vi "AMZ_S3_APIHLP_Multipart Upload Data FG - Get.vi"(8 "error in (no error)":errorcluster, 11 "Multipart Upload RefNum in":T3) -> (0 "error out":errorcluster, 2 "Multipart Upload Data":T1 {"Parts"."PartNumber" min=1 max=10000}, 3 "Multipart Upload RefNum out":T3)   [LabVIEW 2015, in "LV Interface for Amazon S3.lvlib"]
uses:
  LV Interface for Amazon S3.lvlib
  Typedefs/AMZ_S3_Multipart Upload RefNum.ctl
  Typedefs/AMZ_S3_Multipart Upload RefNum Enum.ctl
  Typedefs/AMZ_S3_Multipart Upload Data.ctl
  Typedefs/AMZ_S3_Multipart Upload Part Data.ctl
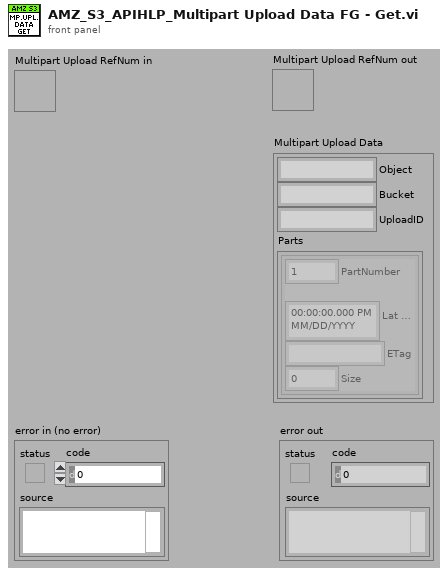
[diagram p1: front panel]
types:
  T1 = typedef "LV Interface for Amazon S3.lvlib/AMZ_S3_Multipart Upload Data.ctl" = cluster{"Object":string, "Bucket":string, "UploadID":string, "Parts":T2[]}
  T2 = typedef "LV Interface for Amazon S3.lvlib/AMZ_S3_Multipart Upload Part Data.ctl" = cluster{"PartNumber":u16, "Lat modified":timestamp, "ETag":string, "Size":u64}
  T3 = typedef "LV Interface for Amazon S3.lvlib/AMZ_S3_Multipart Upload RefNum.ctl" = refnum<k1>
  T4 = typedef "AMZ_S3_Toolkit.lvlib/AMZ_S3_Multipart Upload Data.ctl" = cluster{"Object":string, "Bucket":string, "UploadID":string, "Parts":T5[]}
  T5 = typedef "AMZ_S3_Toolkit.lvlib/AMZ_S3_Multipart Upload Part Data.ctl" = cluster{"PartNumber":u16, "Lat modified":timestamp, "ETag":string, "Size":u64}
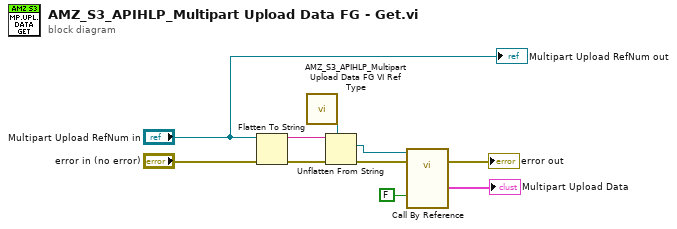
[diagram p0: block diagram]
diagram:
  n1 = Flatten To String(anything="Multipart Upload RefNum in", error in (no error)="error in (no error)") -> (data string=w10:string, error out=w8:errorcluster)  [unwired: 2 in, 1 out]
  n2 = call "AMZ_S3_APIHLP_Multipart Upload Data FG VI Ref Type.vi"() -> ("VI Refnum (Multipart Upload Data FG.vi Type)"=w1:refnum<vi>)
  n3 = Unflatten From String(type=w1, binary string=w10, error in (no error)=w8) -> (value=w6:refnum<vi>, error out=w7:errorcluster)  [unwired: 2 in, 1 out]
  n4 = call-by-ref "?"(reference=w6, error in=w7, "Set?"=FALSE) -> (error out=→"error out":errorcluster, "Multipart Upload Data"=→"Multipart Upload Data":T4)  [unwired: 1 in, 1 out]
  "Multipart Upload RefNum out" <- "Multipart Upload RefNum in"
